vi "gestione menù a tendina.vi"() -> ()   [LabVIEW 2019]
uses:
  Global percorso impostazioni.vi
  <vilib>/Utility/file.llb/Read From Spreadsheet File (string).vi
  <vilib>/Utility/file.llb/Write Delimited Spreadsheet (string).vi
panel:
  in  "Salva modelli":bool
  in  "FAMIGLIA":u16(ring) items=["FAMIGLIA", "GENERATORE", "GENERICO", "MOTORE C.A."]
  in  "Save Button":bool
  out "Elemento rimosso":string
  in  "Togli":bool
  in  "Menù a tendina:":u16(ring) items=["FAMIGLIA", "MODELLO"]
  in  "Inserisci":bool
  in  "exit":bool
  in  "Multicolumn Listbox":i32(listbox)
  in  "Nuovo elemento":string
  # "Nota: Drag and Drop per cambiare la\nposizione degli elementi"
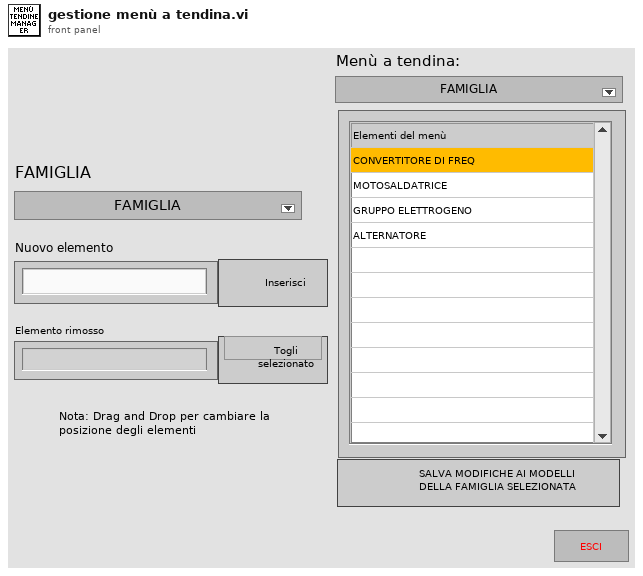
[diagram p1: front panel]
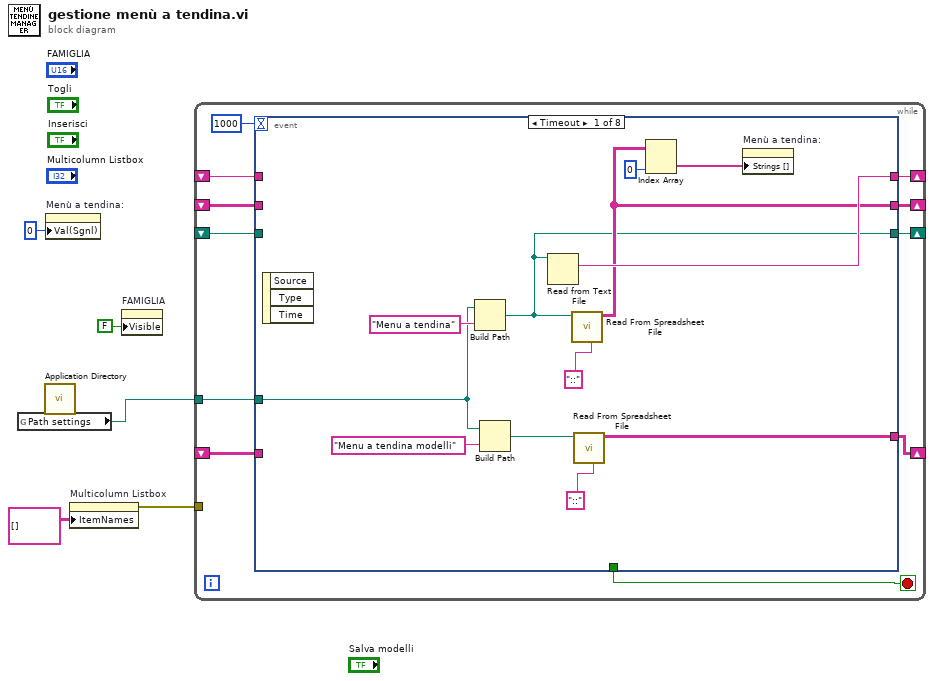
[diagram p0: block diagram]
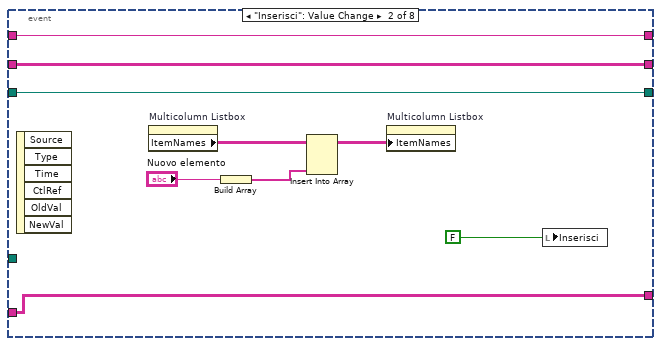
[diagram p2: hidden frame]
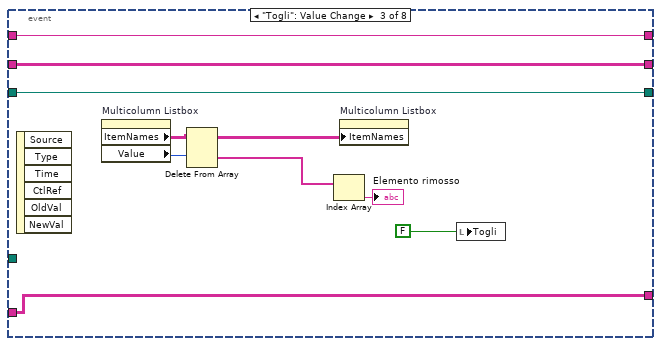
[diagram p3: hidden frame]
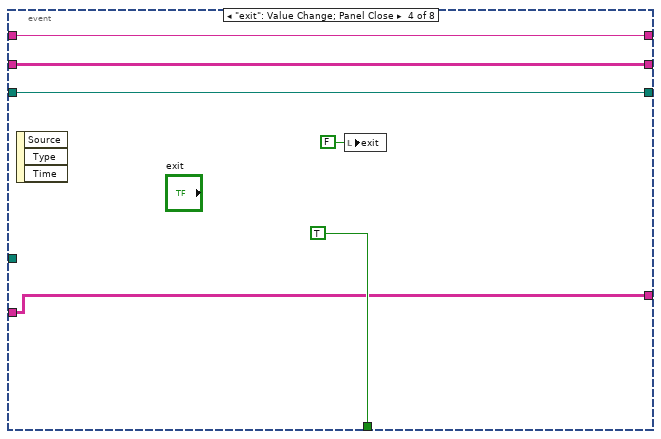
[diagram p4: hidden frame]
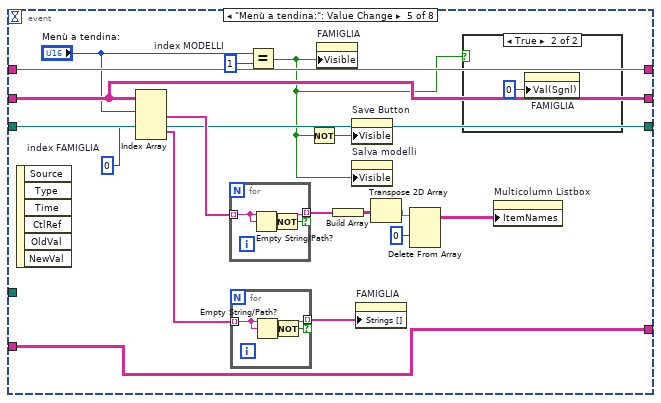
[diagram p5: hidden frame]
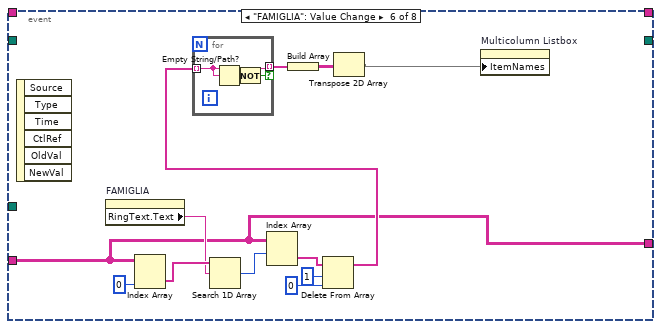
[diagram p7: hidden frame]
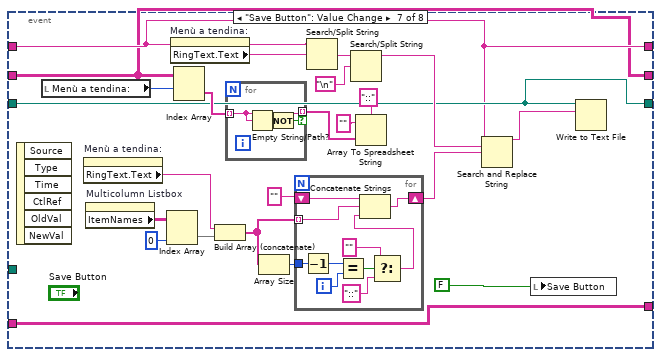
[diagram p8: hidden frame]
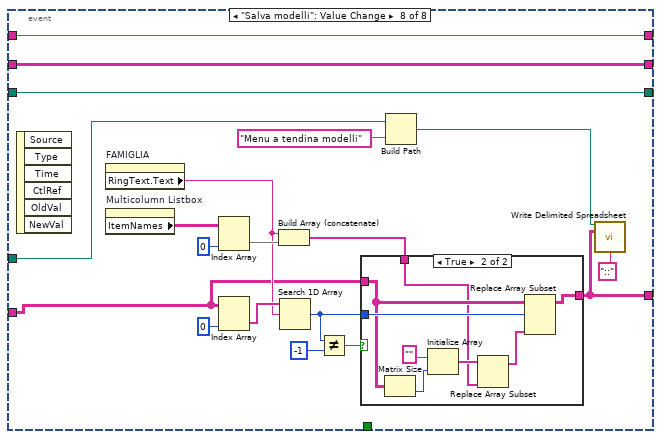
[diagram p9: hidden frame]
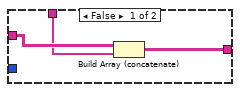
[diagram p10: hidden frame]
diagram:
  n1 = global read "Global percorso impostazioni.vi" "Path settings"() -> (w3:path)
  n2 = call <vilib>:"Application Directory.vi"() -> ()  [unwired: 1 out]
  n3 = property on="Menù a tendina:" class="Ring (strict)"("Val(Sgnl)"=u16 0 ("Value (Signaling)")) -> ()  [unwired: 2 in, 2 out]
  n4 = property on="Multicolumn Listbox" class="MCListbox (strict)"("ItemNames"=string[][] [] ("Item Names")) -> (error out=w2:errorcluster)  [unwired: 2 in, 1 out]
  n5 = property on="FAMIGLIA" class="Ring (strict)"("Visible"=FALSE) -> ()  [unwired: 2 in, 2 out]
  n6 = while {
    shift-right: [w11] -> _
    shift-left: _ -> [w13]
    shift-right: [w10] -> _
    shift-left: _ -> [w15]
    shift-right: [w9] -> _
    shift-left: _ -> [w14]
    shift-right: [w8] -> _
    shift-left: _ -> [w7]
    tunnel: w3 -> [w6]
    tunnel: w2 -> [_]
    stop <- w16 stop-if-true
    n7 = event shown="[0] Timeout" {
      selector: _ -> [_ _ _ _ _ _ _ _]
      dyn-events: _ -> [_ _ _ _ _ _ _ _]
      timeout: 1000 -> [_ _ _ _ _ _ _ _]
      tunnel: [_ _ _ TRUE _ _ _ _] -> w16
      tunnel: w15 -> [_ w31 w40 w52 w63 _ w94 w130]
      tunnel: w14 -> [_ w30 w39 w51 w62 _ w96 w131]
      tunnel: w13 -> [_ w32 w41 w53 w64 _ w95 w129]
      tunnel: [w24 w32 w41 w53 w64 _ w95 w129] -> w11
      tunnel: [w23 w31 w40 w52 w63 _ w94 w130] -> w10
      tunnel: [w22 w30 w39 w51 w62 _ w96 w131] -> w9
      tunnel: [w18 w29 w38 w48 w56 w79 w93 w136] -> w8
      tunnel: w7 -> [_ w29 w38 w48 w56 w79 w93 w141]
      tunnel: w6 -> [w17 _ _ _ _ _ _ w134]
      event Timeout {
        n8 = event-data() -> ()  [unwired: 1 in, 3 out]
        n9 = Build Path(base path=w17, name or relative path="Menu a tendina") -> (appended path=w22:path)
        n10 = Build Path(base path=w17, name or relative path="Menu a tendina modelli") -> (appended path=w19:path)
        n11 = Read from Text File(file (use dialog)=w22) -> (text=w24:string)  [unwired: 3 in, 3 out]
        n12 = call-poly <vilib>:"Read From Spreadsheet File.vi"("delimiter (\\t)"="::" ("delimiter (\\t)"), "file path (dialog if empty)"=w22) -> ("all rows"=w23:string[][])  [unwired: 5 in, 4 out]
        n13 = call-poly <vilib>:"Read From Spreadsheet File.vi"("delimiter (\\t)"="::" ("delimiter (\\t)"), "file path (dialog if empty)"=w19) -> ("all rows"=w18:string[][])  [unwired: 5 in, 4 out]
        n14 = Index Array(array=w23, index (col)=0 ("disabled index (col)")) -> (element=w28:string[])  [unwired: 1 in]
        n15 = property on="Menù a tendina:" class="Ring (strict)"("Strings []"=w28) -> ()  [unwired: 2 in, 2 out]
      }
      event "Inserisci": Value Change {
        n16 = event-data() -> ()  [unwired: 1 in, 6 out]
        n17 = property on="Multicolumn Listbox" class="MCListbox (strict)"() -> ("ItemNames"=w37:string[][])  [unwired: 2 in, 2 out]
        n18 = Build Array("Nuovo elemento") -> (w34:string[])
        n19 = Insert Into Array(array=w37, new element=w34) -> (w36:string[][])  [unwired: 2 in]
        n20 = property on="Multicolumn Listbox" class="MCListbox (strict)"("ItemNames"=w36) -> ()  [unwired: 2 in, 2 out]
        n21 = local write "Inserisci"(FALSE ("Inserisci")) -> ()
      }
      event "Togli": Value Change {
        n22 = event-data() -> ()  [unwired: 1 in, 6 out]
        n23 = property on="Multicolumn Listbox" class="MCListbox (strict)"() -> ("ItemNames"=w47:string[][], "Value"=w45:i32)  [unwired: 2 in, 2 out]
        n24 = Delete From Array(array=w47, index (row)=w45) -> (deleted portion=w44:string[], array with subset deleted=w46:string[][])  [unwired: 2 in]
        n25 = Index Array(array=w44) -> (element=→"Elemento rimosso":string)  [unwired: 1 in]
        n26 = property on="Multicolumn Listbox" class="MCListbox (strict)"("ItemNames"=w46) -> ()  [unwired: 2 in, 2 out]
        n27 = local write "Togli"(FALSE ("Togli")) -> ()
      }
      event "exit": Value Change; Panel Close {
        n28 = event-data() -> ()  [unwired: 1 in, 3 out]
        n29 = local write "exit"(FALSE ("exit")) -> ()
      }
      event "Menù a tendina:": Value Change {
        w57 = u16 1  # index MODELLI
        w61 = 0  # index FAMIGLIA
        n30 = event-data() -> ()  [unwired: 1 in, 6 out]
        n31 = Index Array(array=w63, index (row) #1="Menù a tendina:", index (row) #2=w61) -> (element #1=w66:string[], element #2=w60:string[])  [unwired: 2 in]
        n32 = for {
          tunnel: w66 -> [w77] mode=indexing
          tunnel: [w77] -> w65 mode=indexing if=w75
          n33 = Empty String/Path?(string/path=w77) -> (empty?=w76:bool)
          n34 = Not(x=w76) -> (.not. x?=w75:bool)
        }
        n35 = for {
          tunnel: w60 -> [w74] mode=indexing
          tunnel: [w74] -> w59 mode=indexing if=w72
          n36 = Empty String/Path?(string/path=w74) -> (empty?=w73:bool)
          n37 = Not(x=w73) -> (.not. x?=w72:bool)
        }
        n38 = Equal?(x="Menù a tendina:", y=w57) -> (x = y?=w55:bool)
        n39 = Not(x=w55) -> (.not. x?=w54:bool)
        n40 = property on="FAMIGLIA" class="Ring (strict)"("Visible"=w55) -> ()  [unwired: 2 in, 2 out]
        n41 = Build Array(w65) -> (w70:string[][])
        n42 = property on="Save Button" class="Bool (strict)"("Visible"=w54) -> ()  [unwired: 2 in, 2 out]
        n43 = property on="Salva modelli" class="Bool (strict)"("Visible"=w55) -> ()  [unwired: 2 in, 2 out]
        n44 = property on="FAMIGLIA" class="Ring (strict)"("Strings []"=w59) -> ()  [unwired: 2 in, 2 out]
        n45 = Transpose 2D Array(2D array=w70) -> (transposed array=w69:string[][])
        n46 = Delete From Array(array=w69, index (row)=0) -> (array with subset deleted=w68:string[][])  [unwired: 2 in, 1 out]
        n47 = case shown="True" w55 {
          frame False {
          }
          frame True {
            n48 = property on="FAMIGLIA" class="Ring (strict)"("Val(Sgnl)"=u16 0 ("Value (Signaling)")) -> ()  [unwired: 2 in, 2 out]
          }
        }
        n49 = property on="Multicolumn Listbox" class="MCListbox (strict)"("ItemNames"=w68) -> ()  [unwired: 2 in, 2 out]
      }
      event "FAMIGLIA": Value Change {
        n50 = event-data() -> ()  [unwired: 1 in, 6 out]
        n51 = property on="FAMIGLIA" class="Ring (strict)"() -> ("RingText.Text"=w87:string)  [unwired: 2 in, 2 out]
        n52 = Index Array(array=w79, index (col)=0 ("disabled index (col)")) -> (element=w88:string[])  [unwired: 1 in]
        n53 = Search 1D Array(1D array=w88, element=w87) -> (index of element=w86:i32)  [unwired: 1 in]
        n54 = Index Array(array=w79, index (row)=w86) -> (element=w85:string[])  [unwired: 1 in]
        n55 = Delete From Array(array=w85, length=1, index=0) -> (array with subset deleted=w80:string[])  [unwired: 1 out]
        n56 = for {
          tunnel: w80 -> [w92] mode=indexing
          tunnel: [w92] -> w81 mode=indexing if=w90
          n57 = Empty String/Path?(string/path=w92) -> (empty?=w91:bool)
          n58 = Not(x=w91) -> (.not. x?=w90:bool)
        }
        n59 = Build Array(w81) -> (w82:string[][])
        n60 = Transpose 2D Array(2D array=w82) -> (transposed array=w78:string[][])
        n61 = property on="Multicolumn Listbox" class="MCListbox (strict)"("ItemNames"=w78) -> ()  [unwired: 2 in, 2 out]
      }
      event "Save Button": Value Change {
        n62 = event-data() -> ()  [unwired: 1 in, 6 out]
        n63 = local read "Menù a tendina:"() -> (w115:u16)
        n64 = property on="Menù a tendina:" class="Ring (strict)"() -> ("RingText.Text"=w109:string)  [unwired: 2 in, 2 out]
        n65 = property on="Multicolumn Listbox" class="MCListbox (strict)"() -> ("ItemNames"=w112:string[][])  [unwired: 2 in, 2 out]
        n66 = Index Array(array=w112, index (col)=0 ("disabled index (col)")) -> (element=w110:string[])  [unwired: 1 in]
        n67 = property on="Menù a tendina:" class="Ring (strict)"() -> ("RingText.Text"=w104:string)  [unwired: 2 in, 2 out]
        n68 = Index Array(array=w94, index (row)=w115) -> (element=w107:string[])  [unwired: 1 in]
        n69 = Build Array (concatenate)(w109, w110) -> (w99:string[])
        n70 = for {
          tunnel: w107 -> [w128] mode=indexing
          tunnel: [w128] -> w106 mode=indexing if=w126
          n71 = Empty String/Path?(string/path=w128) -> (empty?=w127:bool)
          n72 = Not(x=w127) -> (.not. x?=w126:bool)
        }
        n73 = Array Size(array=w99) -> (size(s)=w98:i32)
        n74 = for {
          tunnel: w99 -> [w123] mode=indexing
          shift-right: [w125] -> w100
          shift-left: "" -> [w124]
          tunnel: w98 -> [w121]
          i -> [w122]
          n75 = Decrement(x=w121) -> (x-1=w116:i32)
          n76 = Equal?(x=w116, y=w122) -> (x = y?=w120:bool)
          n77 = Select(t="", s=w120, f="::" ("string")) -> (s? t:f=w118:string)
          n78 = Concatenate Strings(w124, w123, w118) -> (w125:string)
        }
        n79 = Search/Split String(string=w95, search string/char (-)=w104) -> (match + rest of string=w105:string)  [unwired: 1 in, 2 out]
        n80 = Search/Split String(string=w105, search string/char (-)="\n") -> (substring before match=w102:string)  [unwired: 1 in, 2 out]
        n81 = Array To Spreadsheet String(delimiter (Tab)="::", array=w106, 3:"" ("format string")) -> ()  [unwired: 1 out]
        n82 = Search and Replace String(input string=w95, search string=w102, replace string=w100) -> (result string=w108:string)  [unwired: 5 in, 3 out]
        n83 = local write "Save Button"(FALSE ("Save Button")) -> ()
        n84 = Write to Text File(file (use dialog)=w96, text=w108) -> ()  [unwired: 2 in, 3 out]
      }
      event "Salva modelli": Value Change {
        n85 = event-data() -> ()  [unwired: 1 in, 6 out]
        n86 = property on="FAMIGLIA" class="Ring (strict)"() -> ("RingText.Text"=w142:string)  [unwired: 2 in, 2 out]
        n87 = property on="Multicolumn Listbox" class="MCListbox (strict)"() -> ("ItemNames"=w147:string[][])  [unwired: 2 in, 2 out]
        n88 = Index Array(array=w147, index (col)=0 ("disabled index (col)")) -> (element=w145:string[])  [unwired: 1 in]
        n89 = Index Array(array=w141, index (col)=0 ("disabled index (col)")) -> (element=w143:string[])  [unwired: 1 in]
        n90 = Build Array (concatenate)(w142, w145) -> (w140:string[])
        n91 = Search 1D Array(1D array=w143, element=w142) -> (index of element=w139:i32)  [unwired: 1 in]
        n92 = Not Equal?(x=w139, y=-1) -> (x != y?=w137:bool)
        n93 = case shown="True" w137 {
          tunnel: w141 -> [w150 w156]
          tunnel: w139 -> [_ w158]
          tunnel: w140 -> [w149 w152]
          tunnel: [w148 w157] -> w136
          frame False {
            n94 = Build Array (concatenate)(w150, w149) -> (w148:string[][])
          }
          frame True {
            n95 = Matrix Size(0:w156) -> (2:w155:i32)  [unwired: 1 out]
            n96 = Initialize Array("", w155) -> (w153:string[])
            n97 = Replace Array Subset(array=w153, new element=w152) -> (w151:string[])  [unwired: 1 in]
            n98 = Replace Array Subset(array=w156, new element=w151, index (row)=w158) -> (w157:string[][])  [unwired: 1 in]
          }
        }
        n99 = Build Path(base path=w134, name or relative path="Menu a tendina modelli") -> (appended path=w132:path)
        n100 = call-poly <vilib>:"Write Delimited Spreadsheet.vi"("file path (dialog if empty)"=w132, "2D data"=w136, "delimiter (\\t)"="::" ("delimiter (\\t)")) -> ()  [unwired: 11 in, 2 out]
      }
    }
  }
